vi "Get Status.vi"(8 "error in (no error)":errorcluster, 11 "Person In":refnum<class "Person.lvclass">) -> (0 "error out":errorcluster, 2 "Status":string, 3 "Person Out":refnum<class "Person.lvclass">)   [LabVIEW 2020, in "Person.lvclass"]
uses:
  Person.lvclass
  C:/Program Files (x86)/National Instruments/LabVIEW 2020/vi.lib/Astemes/Triarc Framework/Process/Process.lvclass
  <vilib>/Astemes/Triarc Framework/Process/Process.lvclass/Process.ctl
  <vilib>/Astemes/Triarc Framework/Synchronous Request Callback/Synchronous Request Callback.lvclass/Synchronous Request Callback.ctl
  Person.lvclass/Person.ctl
  <vilib>/Utility/error.llb/Clear Errors.vi
  <vilib>/Astemes/Triarc Framework/Synchronous Request Callback/Create.vi
  <vilib>/Astemes/Triarc Framework/Process/Protected/Messaging/Async Request Message.vi
  <vilib>/Astemes/Triarc Framework/Process/Private/SubVIs/Handle Debug Data.vi
  <vilib>/Astemes/Triarc Framework/Logging/Log Debug.vi
  <vilib>/AdvancedString/1D String Array to Delimited String.vi
  <vilib>/Utility/High Resolution Relative Seconds.vi
  <vilib>/Astemes/Triarc Framework/Synchronous Request Callback/Synchronous Request Callback.lvclass
  C:/Program Files (x86)/National Instruments/LabVIEW 2020/vi.lib/Astemes/Triarc Framework/Callback/Callback.lvclass
  <vilib>/Astemes/Triarc Framework/Process/Process.lvclass
  C:/Program Files (x86)/National Instruments/LabVIEW 2020/vi.lib/Astemes/Triarc Framework/Logging/Logging.lvclass
  <vilib>/Utility/error.llb/Error Cluster From Error Code.vi
  <vilib>/Astemes/Triarc Framework/Process/Public/Read Name.vi
  <vilib>/Astemes/Triarc Framework/Process/Private/SubVIs/Wait for Response Message.vi
  <vilib>/Astemes/Triarc Framework/Callback/Callback.lvclass
  <vilib>/Astemes/Triarc Framework/Logging/Logging.lvclass
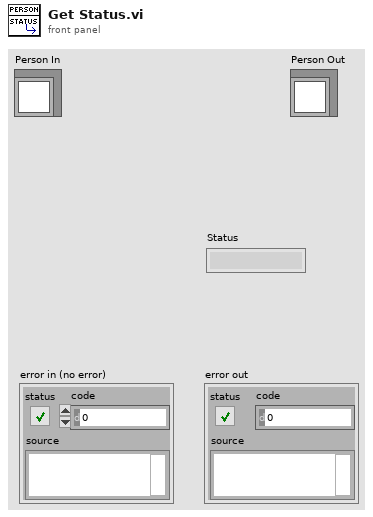
[diagram p1: front panel]
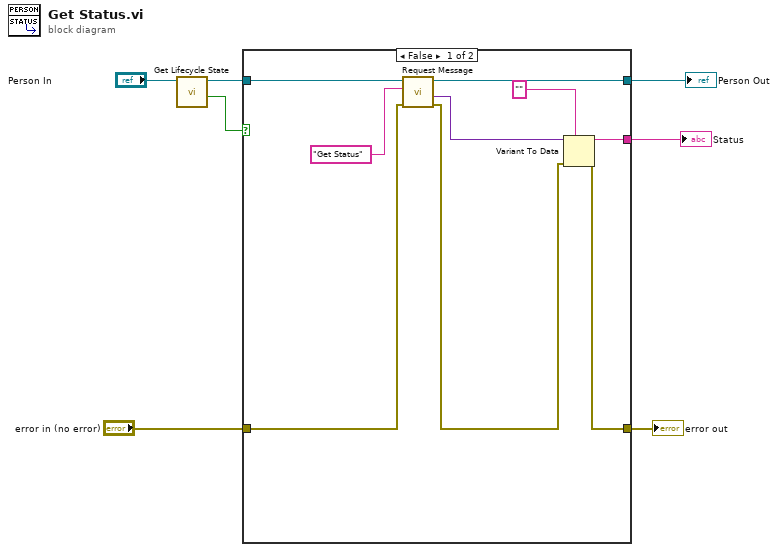
[diagram p0: block diagram]
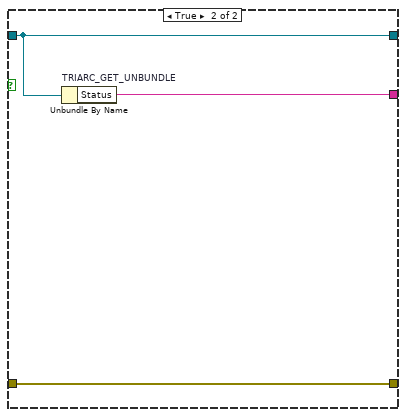
[diagram p2: hidden frame]
diagram:
  n1 = call <vilib>:"Get Lifecycle State.vi"("Process In"="Person In") -> ("In Process Loop?"=w2:bool, "Process Out"=w6:refnum<class "Person.lvclass">)  [unwired: 7 in, 2 out]
  n2 = case shown="False" w2 {
    tunnel: w6 -> [w16 w19]
    tunnel: [w15 w19] -> w5
    tunnel: "error in (no error)" -> [w14 w18]
    tunnel: [w11 w18] -> w4
    tunnel: [w9 w17] -> w3
    frame False {
      n3 = call <vilib>:"Request Message.vi"("error in (no error)"=w14, "Request Message"="Get Status" ("API Message"), "Process In"=w16) -> ("error out"=w12:errorcluster, "Response Message Data"=w13:variant, "Process Out"=w15:refnum<class "Person.lvclass">)  [unwired: 4 in, 2 out]
      n4 = Variant To Data(error in=w12, type="" ("Type Speifier"), Variant=w13) -> (data=w9:string, error out=w11:errorcluster)
    }
    frame True {
      n5 = Unbundle By Name "TRIARC_GET_UNBUNDLE"(w19) -> ("Status"=w17:string)
    }
  }
  "error out" <- w4
  "Person Out" <- w5
  "Status" <- w3
